vi "标记特殊单元格.vi"() -> ()   [LabVIEW 2013, in "Table Tool.lvlib"]
uses:
  Table Tool.lvlib
panel:
  in  "阙值":dbl=0.8
  in  "Normal":u32(colorbox)=16448250
  in  "Mark":u32(colorbox)=16711680
  in  "停止按钮":bool
  out "随机数":string[][](table)=[["0.588590", "0.481400", "0.701046"], ["0.967495", "0.280380", "0.824204"], ["0.758888", "0.777537", "0.967250"], ["0.180166", "0.980441", "0.547606"], ["0.886610", "0.445899", "0.280210"], ["0.719594", "0.385798", "0.299601"], ["0.747303", "0.522431", "0.814879"], ["0.506352", "0.321613", "0.651681"], ["0.168636", "0.117135", "0.068814"], ["0.855561", "0.657755", "0.671170"], ["0.424404", "0.584779", "0.427216"], ["0.223649", "0.298725", "0.850261"], ["0.740891", "0.425520", "0.501349"], ["0.150256", "0.297018", "0.084259"], ["0.301690", "0.732232", "0.761721"], ["0.001024", "0.426565", "0.283347"], ["0.483586", "0.628862", "0.571545"], ["0.627284", "0.001871", "0.009066"], ["0.610636", "0.168952", "0.784596"], ["0.250156", "0.506958", "0.442624"]]
  in  "列数":i32=3
  in  "行数":i32=20
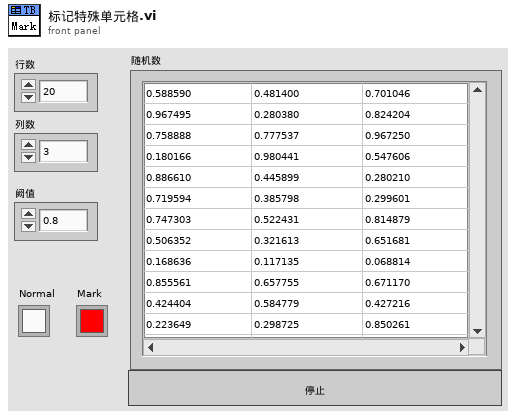
[diagram p1: front panel]
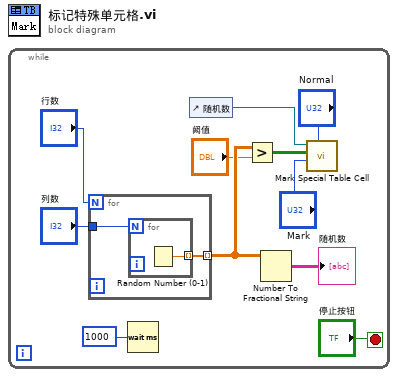
[diagram p0: block diagram]
diagram:
  n1 = while {
    stop <- "停止按钮" stop-if-true
    n2 = for {
      N: "行数" -> [_]
      tunnel: "列数" -> [w13]
      tunnel: [w12] -> w9 mode=indexing
      n3 = for {
        N: w13 -> [_]
        tunnel: [w14] -> w12 mode=indexing
        n4 = Random Number (0-1)() -> (number: 0 to 1=w14:dbl)
      }
    }
    n5 = Wait (ms)(milliseconds to wait=u32 1000 ("等待时间（毫秒）")) -> ()  [unwired: 1 out]
    n6 = control-ref of="随机数"() -> (w6:refnum<vi>)
    n7 = Greater?(x=w9, y="阙值") -> (0:w7:bool[][])
    n8 = Number To Fractional String(number=w9) -> (F-format string=→"随机数":string[][])  [unwired: 3 in]
    n9 = call "Mark Special Table Cell.vi"("Normal"="Normal", "Mark"="Mark", "Mark Array"=w7, "Table Ref In"=w6) -> ()  [unwired: 6 in, 2 out]
  }
